vi "hind brain 3.vi"() -> ()   [LabVIEW 2011, in "Hindbrain Demo.lvrbt"]
uses:
  Hindbrain Demo.lvrbt
  <vilib>/NXT/Subs/LVHSConnector.ctl
  <vilib>/NXT/Block Support/HWPage.SensorType.ctl
  <vilib>/NXT/Block Support/HWPage.SensorMode.ctl
  <vilib>/NXT/Block Support/NXT_InputPort.ctl
  <vilib>/addons/mindsensors.com_LVEE_Toolkit_V1.23/mindsensors.com LVEE Toolkit/Dual/Distance Sensor-DM.vi
  <vilib>/addons/mindsensors.com_LVEE_Toolkit_V1.23/mindsensors.com LVEE Toolkit/Dual/NXTServo-DM.vi
  <vilib>/NXT/Dual Mode Library/Sensors/Color_None.vi
panel:
  in  "stop 2":bool
  out "NXT dup":T1={"Hardware"="NXT", "Flattened String"=""} caption="NXT"
  in  "Input of NXTServo 2":T2={"Servo Number"=2, "Position"=1500, "Speed"=0} {"Speed" step=1 scale=0.0..255.0; "Position" min=500 max=2500 step=1 scale=500.0..2500.0; "Servo Number" min=1 max=8 step=1}
  out "Output of NXTServo 2":cluster{"Voltage":u8, "Status":bool}
  in  "stop":bool
  in  "Input of NXTServo":T2={"Servo Number"=1, "Position"=1500, "Speed"=0} {"Speed" step=1 scale=0.0..255.0; "Position" min=500 max=2500 step=1 scale=500.0..2500.0; "Servo Number" min=1 max=8 step=1}
  out "Output of NXTServo":cluster{"Voltage":u8, "Status":bool}
  out "Pressed?":bool caption="Switch\nPressed?"
  out "Light Intensity":i16 caption="Scaled Value"
  out "Blink":bool
  out "Battery mv":i32
  out "Scaled Value":i16
  out "Left?":bool
  out "Right?":bool
  out "Front?":bool
  out "Stuff?":bool
  # "This is a demonstration of how to sense and acturate devices on the LEGO NXT brick.\nThe connections to the NXT brick are as follows:\nNOTHING IS CONNECTED TO PORTS A, B AND C.\nPort 1 has the Mindsensor NXTServo\nPort 2 has the LEGO Color Sensor\nPort 3 has the LEGO Switch\nPort 4 and the Mindsensor NXTSumoEyes-v3."
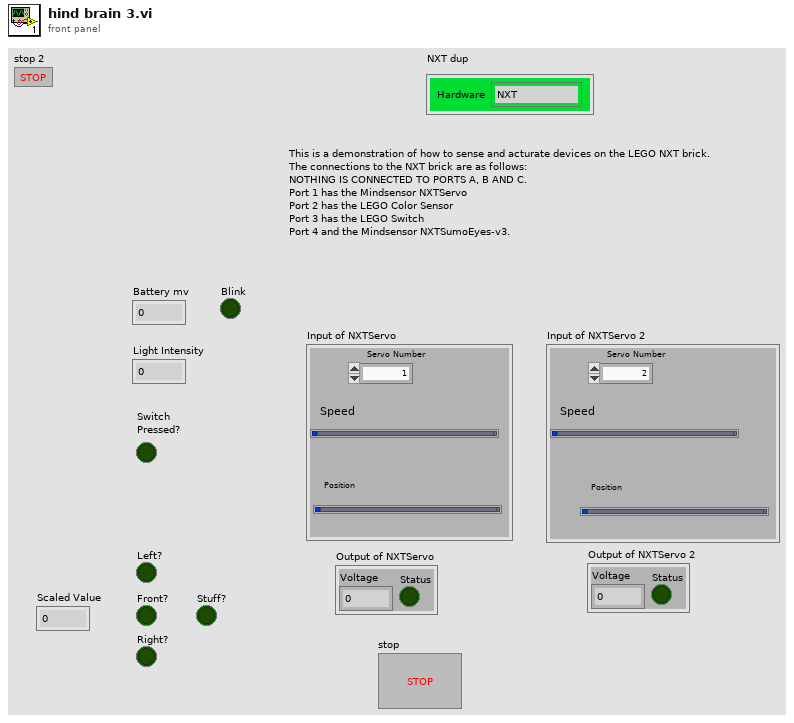
[diagram p1: front panel]
types:
  T1 = typedef "LVHSConnector.ctl" = cluster{"Hardware":string, "Flattened String":string}
  T2 = cluster{"Servo Number":u8, "Position":u16, "Speed":u8}
  T3 = typedef "NXT_InputPort.ctl" = u8
  T4 = typedef "HWPage.SensorType.ctl" = u8
  T5 = typedef "HWPage.SensorMode.ctl" = u8
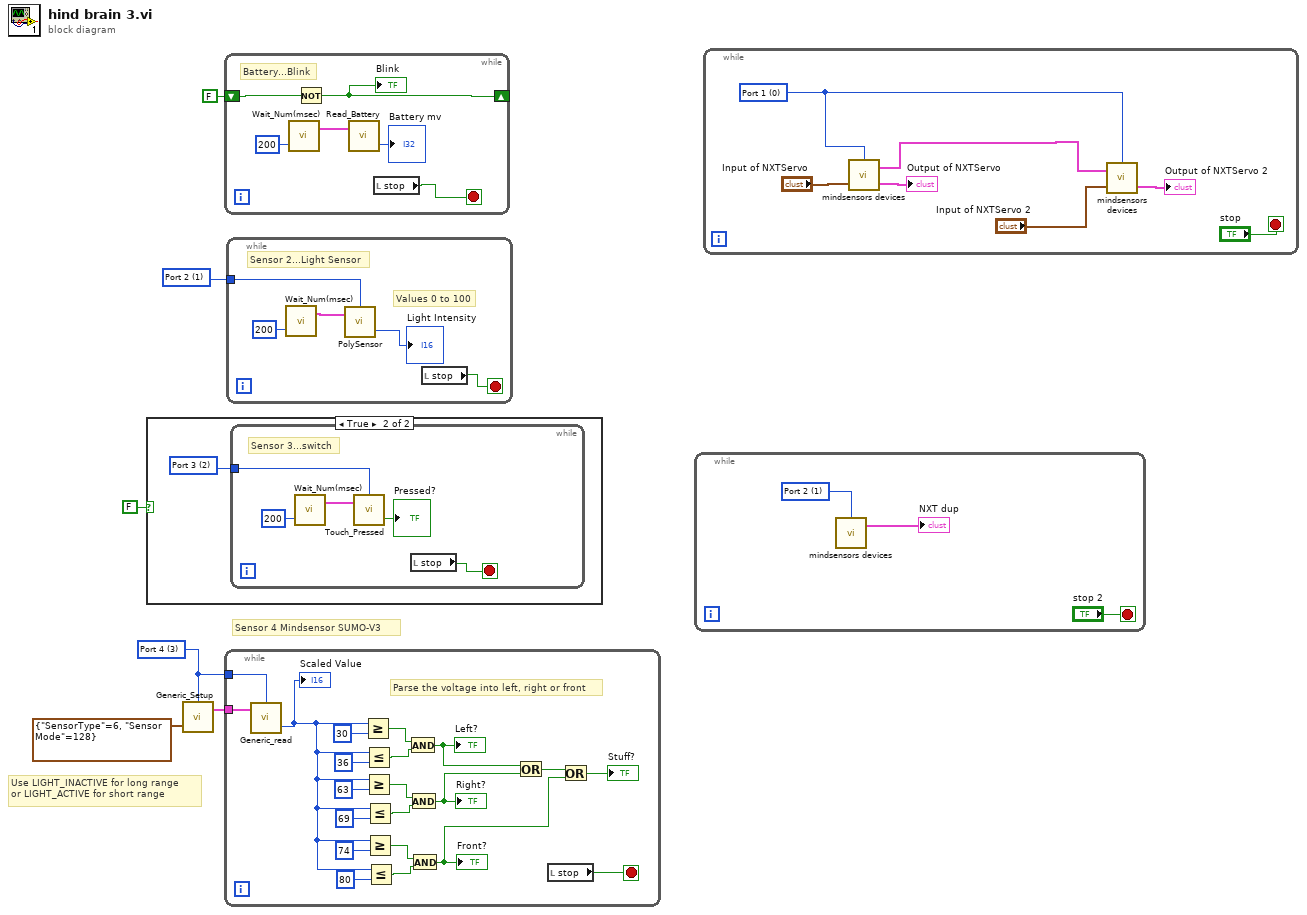
[diagram p0: block diagram]
diagram:
  w2 = T3 1 items=["Port 1", "Port 2", "Port 3", "Port 4"] ("Port (Port 3)")
  w3 = T3 3 items=["Port 1", "Port 2", "Port 3", "Port 4"] ("Port")
  # "Sensor 4 Mindsensor SUMO-V3"
  # "Use LIGHT_INACTIVE for long range\nor LIGHT_ACTIVE for short range"
  n1 = case shown="True" FALSE {
    frame False {
    }
    frame True {
      w7 = T3 2 items=["Port 1", "Port 2", "Port 3", "Port 4"] ("Port (Port 1)")
      n2 = while {
        tunnel: w7 -> [w9]
        stop <- w10 stop-if-true
        # "Sensor 3...switch"
        n3 = call <vilib>:"Wait_Num(msec).vi"("Time (100 msec)"=u32 200) -> ("NXT"=w11:T1)  [unwired: 3 in]
        n4 = call <vilib>:"Touch_Pressed.vi"("NXT"=w11, "Port (Port 1)"=w9) -> ("Yes / No"=→"Pressed?":bool)  [unwired: 1 in, 1 out]
        n5 = local read "stop"() -> (w10:bool)
      }
    }
  }
  n6 = call <vilib>:"Generic_Setup.vi"("Sensor Setup"=cluster{"SensorType":T4, "Sensor Mode":T5} {"SensorType"=6, "Sensor Mode"=128}, "Port"=w3) -> ("NXT"=w6:T1)  [unwired: 1 in, 1 out]
  n7 = while {
    shift-right: [w14] -> _
    shift-left: FALSE -> [w15]
    stop <- w16 stop-if-true
    # "Battery...Blink"
    n8 = call <vilib>:"Wait_Num(msec).vi"("Time (100 msec)"=u32 200) -> ("NXT"=w17:T1)  [unwired: 3 in]
    n9 = Not(x=w15) -> (.not. x?=w14:bool)
    "Blink" <- w14
    n10 = call <vilib>:"Read_Battery.vi"("NXT"=w17) -> ("millivolts"=→"Battery mv":i32)  [unwired: 2 in, 1 out]
    n11 = local read "stop"() -> (w16:bool)
  }
  n12 = while {
    tunnel: w3 -> [w39]
    tunnel: w6 -> [w38]
    stop <- w19 stop-if-true
    # "Parse the voltage into left, right or front"
    n13 = call <vilib>:"Generic_read.vi"("NXT"=w38, "Port (Port 3)"=w39) -> ("Scaled Value"=w25:i16)  [unwired: 2 out]
    "Scaled Value" <- w25
    n14 = Greater Or Equal?(x=w25, y=i16 30) -> (x >= y?=w35:bool)
    n15 = Less Or Equal?(x=w25, y=i16 36) -> (x <= y?=w34:bool)
    n16 = Greater Or Equal?(x=w25, y=i16 63) -> (x >= y?=w32:bool)
    n17 = Less Or Equal?(x=w25, y=i16 69) -> (x <= y?=w33:bool)
    n18 = Greater Or Equal?(x=w25, y=i16 74) -> (x >= y?=w28:bool)
    n19 = Less Or Equal?(x=w25, y=i16 80) -> (x <= y?=w29:bool)
    n20 = And(x=w35, y=w34) -> (x .and. y?=w24:bool)
    "Left?" <- w24
    n21 = And(x=w32, y=w33) -> (x .and. y?=w23:bool)
    "Right?" <- w23
    n22 = And(x=w28, y=w29) -> (x .and. y?=w21:bool)
    "Front?" <- w21
    n23 = Or(x=w24, y=w23) -> (x .or. y?=w22:bool)
    n24 = local read "stop"() -> (w19:bool)
    n25 = Or(x=w22, y=w21) -> (x .or. y?=→"Stuff?":bool)
  }
  n26 = while {
    tunnel: w2 -> [w40]
    stop <- w43 stop-if-true
    # "Values 0 to 100"
    # "Sensor 2...Light Sensor"
    n27 = call <vilib>:"Wait_Num(msec).vi"("Time (100 msec)"=u32 200) -> ("NXT"=w42:T1)  [unwired: 3 in]
    n28 = call-poly <vilib>:"PolySensor.vi"("NXT"=w42, "Port (Port 3)"=w40) -> ("Intensity"=→"Light Intensity":i16)  [unwired: 1 in, 1 out]
    n29 = local read "stop"() -> (w43:bool)
  }
  n30 = while {
    stop <- "stop 2" stop-if-true
    w47 = T3 1 items=["Port 1", "Port 2", "Port 3", "Port 4"] ("Input Port")
    n31 = call-poly <vilib>:"mindsensors devices.vi"("Input Port"=w47) -> ("NXT dup"=→"NXT dup":T1)  [unwired: 2 in, 1 out]
  }
  n32 = while {
    stop <- "stop" stop-if-true
    w48 = T3 0 items=["Port 1", "Port 2", "Port 3", "Port 4"] ("Input Port")
    n33 = call-poly <vilib>:"mindsensors devices.vi"("Input of NXTServo"="Input of NXTServo", "Input Port"=w48) -> ("Output of NXTServo"=→"Output of NXTServo":cluster{"Voltage":u8, "Status":bool}, "NXT dup"=w49:T1)  [unwired: 1 in]
    n34 = call-poly <vilib>:"mindsensors devices.vi"("Input of NXTServo"="Input of NXTServo 2", "NXT"=w49, "Input Port"=w48) -> ("Output of NXTServo"=→"Output of NXTServo 2":cluster{"Voltage":u8, "Status":bool})  [unwired: 1 out]
  }
